vi "Start Module.vi"(8 "error in (no error)":errorcluster) -> (0 "error out":errorcluster, 1 "Wait for Event Sync?":bool, 2 "PF_trial_1 Broadcast Events":T1, 3 "Module Was Already Running?":bool)   [LabVIEW 2019, in "PF_trial_1.lvlib"]
doc: "Launches the Module Main.vi.\n_____\nBased on Delacor QMH Project Template 5.0.0.82."
uses:
  PF_trial_1.lvlib
  Broadcast Events--cluster.ctl
  Did Init Argument--cluster.ctl
  Status Updated Argument--cluster.ctl
  Error Reported Argument--cluster.ctl
  Stop Argument--cluster.ctl
  Get Module Execution Status Argument--cluster.ctl
  COM PORT Argument--cluster.ctl
  <vilib>/Delacor/Delacor QMH/Libraries/Module Admin_class/Delacor_lib_QMH_Module Admin.lvclass
  <vilib>/Delacor/Delacor QMH/Libraries/Module Admin_class/Delacor_lib_QMH_Module Admin.lvclass/Delacor_lib_QMH_Module Admin.ctl
  <vilib>/Delacor/Delacor QMH/Libraries/Module Admin_class/Delacor_lib_QMH_Set External Launch.vi
  <vilib>/Utility/error.llb/Error Cluster From Error Code.vi
  <vilib>/ErrorRing/Error Ring.xnode
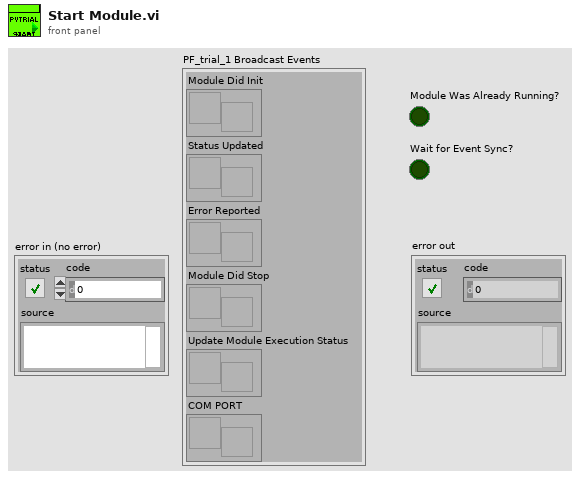
[diagram p1: front panel]
types:
  T1 = typedef "PF_trial_1.lvlib/Broadcast Events--cluster.ctl" = cluster{"Module Did Init":refnum<user-event>, "Status Updated":refnum<user-event>, "Error Reported":refnum<user-event>, "Module Did Stop":refnum<user-event>, "Update Module Execution Status":refnum<user-event>, "COM PORT":refnum<user-event>}
  T2 = enum32{"Bad", "Idle", "Run top level", "Running"}
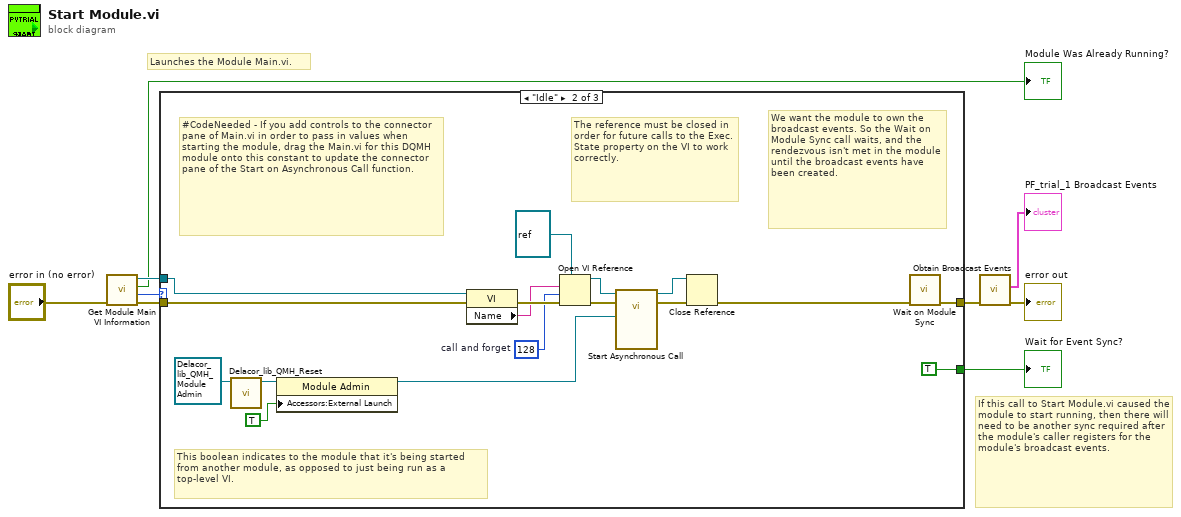
[diagram p0: block diagram]
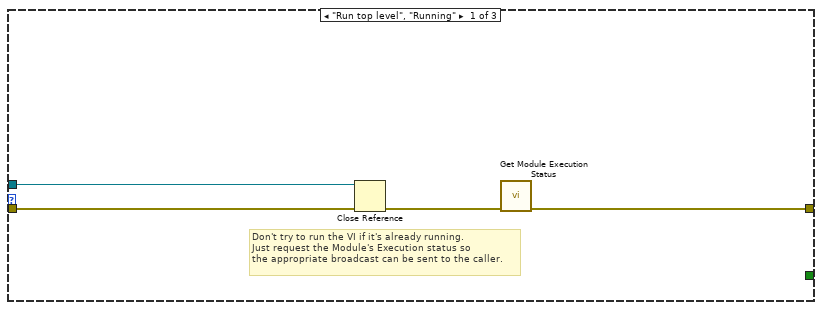
[diagram p2: hidden frame]
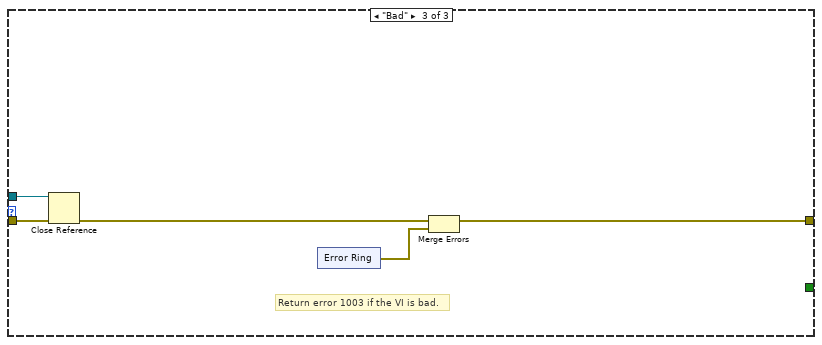
[diagram p3: hidden frame]
diagram:
  # "If this call to Start Module.vi caused the module to start running, then there will need to be another sync required after the module's caller registers for the module's broadcast events."
  # "Launches the Module Main.vi."
  n1 = call "Get Module Main VI Information.vi"("error in (no error)"="error in (no error)") -> ("error out"=w8:errorcluster, "Execution State"=w3:T2, "Is Module Running?"=→"Module Was Already Running?":bool, "Module Main VI"=w7:refnum<vi>)  [unwired: 7 in]
  n2 = case shown="\"Idle\"" w3 {
    tunnel: w8 -> [w13 w30 w35]
    tunnel: w7 -> [w12 w24 w34]
    tunnel: [w10 w29 w32] -> w6
    tunnel: [_ TRUE _] -> w4
    frame "Run top level", "Running" {
      # "Don't try to run the VI if it's already running.\nJust request the Module's Execution status so\nthe appropriate broadcast can be sent to the caller."
      n3 = Close Reference(reference=w12, error in (no error)=w13) -> (error out=w11:errorcluster)
      n4 = call "Get Module Execution Status.vi"("error in (no error)"=w11) -> ("error out"=w10:errorcluster)  [unwired: 10 in]
    }
    frame "Idle" {
      w21 = 128  # call and forget
      # "#CodeNeeded - If you add controls to the connector pane of Main.vi in order to pass in values when starting the module, drag the Main.vi for this DQMH module onto this constant to update the connector pane of the Start on Asynchronous Call function."
      # "The reference must be closed in order for future calls to the Exec.State property on the VI to work correctly."
      # "We want the module to own the broadcast events. So the Wait on Module Sync call waits, and the rendezvous isn't met in the module until the broadcast events have been created."
      # "This boolean indicates to the module that it's being started from another module, as opposed to just being run as a top-level VI."
      n5 = call-dynamic "Delacor_lib_QMH_Reset.vi"("Mod Admin in"=refnum<class "Delacor_lib_QMH_Module Admin.lvclass"> refnum) -> ("Mod Admin out"=w27:refnum<class "Delacor_lib_QMH_Module Admin.lvclass">)  [unwired: 9 in, 1 out]
      n6 = property class="Module Admin"(reference=w27, "Accessors:External Launch"=TRUE) -> (reference out=w18:refnum<class "Delacor_lib_QMH_Module Admin.lvclass">)  [unwired: 1 in, 1 out]
      n7 = property class="VI"(reference=w24, error in=w30) -> (error out=w23:errorcluster, "Name"=w14:string)  [unwired: 1 out]
      n8 = Open VI Reference(type specifier VI Refnum (for type only)=refnum<vi> refnum, vi path=w14, options=w21, error in (no error)=w23) -> (vi reference=w19:refnum<vi>, error out=w20:errorcluster)  [unwired: 2 in]
      n9 = call-by-ref "Start Asynchronous Call"(reference=w19, error in=w20, "Module Admin"=w18) -> (reference out=w16:refnum<vi>, error out=w17:errorcluster)  [unwired: 11 in]
      n10 = Close Reference(reference=w16, error in (no error)=w17) -> (error out=w15:errorcluster)
      n11 = call "Wait on Module Sync.vi"("error in (no error)"=w15) -> ("error out"=w29:errorcluster)  [unwired: 10 in]
    }
    frame "Bad" {
      # "Return error 1003 if the VI is bad."
      n12 = Close Reference(reference=w34, error in (no error)=w35) -> (error out=w33:errorcluster)
      n13 = xnode "Error Ring"() -> ("error out"=w31:errorcluster)
      n14 = Merge Errors(w33, w31) -> (w32:errorcluster)
    }
  }
  "Wait for Event Sync?" <- w4
  n15 = call "Obtain Broadcast Events.vi"("error in (no error)"=w6) -> ("error out"=→"error out":errorcluster, "PF_trial_1 Broadcast Events"=→"PF_trial_1 Broadcast Events":T1)  [unwired: 9 in]
